vi "Telescope Read Current Status.vi"(8 "error in (no error)":errorcluster, 11 "LDT Telescope in":refnum<class "LDT Telescope.lvclass">) -> (0 "error out":errorcluster, 1 "Raw Response":string="TCS.TCSSharedVariables.TCSHighLevelStatusSV.TCSTcsStatusSV\n<tcsTCSStatus>\n  <tcsVersion>V1.9</tcsVersion>\n  <accessMode>Operator</accessMode>\n  <azCurrentWrap>-1</azCurrentWrap>\n  <heartbeat>15339</heartbeat>\n  <inPositionIsTrue>true</inPositionIsTrue>\n  <m1CoverState>Closed</m1CoverState>\n  <mountGuideMode>OpenLoop</mountGuideMode>\n  <rotCurrentWrap>-1</rotCurrentWrap>\n  <tcsHealth>BAD</tcsHealth>\n  <tcsState>ENABLED</tcsState>\n  <currentTimes>\n    <lst>\n      <hours>22</hours>\n      <minutesTime>32</minutesTime>\n      <secondsTime>33.4</secondsTime>\n    </lst>\n    <time>2023-03-24T17:50:28.166+00:00</time>\n  </currentTimes>\n  <limits>\n    <moonProximity>\n      <distance_deg>85.538145066048</distance_deg>\n      <proximityFlag>false</proximityFlag>\n    </moonProximity>\n    <sunProximity>\n      <distance_deg>101.25098674051</distance_deg>\n      <proximityFlag>false</proximityFlag>\n    </sunProximity>\n    <zenith>\n      <currentZD_deg>66.0067</currentZD_deg>\n      <elZenithLimit_deg>89.3</elZenithLimit_deg>\n      <inBlindSpotIsTrue>false</inBlindSpotIsTrue>\n      <timeToBlindSpot_min>-1</timeToBlindSpot_min>\n      <timeToBlindSpotExit_min>-1</timeToBlindSpotExit_min>\n    </zenith>\n    <airmass>2.4476733769952</airmass>\n    <currentTimeToObservable_min>-1</currentTimeToObservable_min>\n    <currentTimeToUnobservable_min>-1</currentTimeToUnobservable_min>\n    <timeToRotLimit_min>-1</timeToRotLimit_min>\n    <timeToAzLimit_min>-1</timeToAzLimit_min>\n  </limits>\n  <pointingPositions>\n    <azElError>\n      <azError>-0.162</azError>\n      <elError>0.09</elError>\n    </azElError>\n    <currentAzEl>\n      <azimuth>\n        <degreesArc>351</degreesArc>\n        <minutesArc>20</minutesArc>\n        <secondsArc>38.2</secondsArc>\n      </azimuth>\n      <elevation>\n        <degreesAlt>23</degreesAlt>\n        <minutesArc>59</minutesArc>\n        <secondsArc>35.9</secondsArc>\n      </elevation>\n    </currentAzEl>\n    <currentHA>\n      <hours>9</hours>\n      <minutesTime>35</minutesTime>\n      <secondsTime>52.01</secondsTime>\n    </currentHA>\n    <currentRADec>\n      <declination>\n        <degreesDec>77</degreesDec>\n        <minutesArc>5</minutesArc>\n        <secondsArc>36.1</secondsArc>\n      </declination>\n      <equinoxPrefix>J</equinoxPrefix>\n      <equinoxYear>2000</equinoxYear>\n      <frame>FK5</frame>\n      <ra>\n        <hours>12</hours>\n        <minutesTime>55</minutesTime>\n        <secondsTime>53.37</secondsTime>\n      </ra>\n    </currentRADec>\n    <currentParAngle>31.951973490925</currentParAngle>\n    <currentRotatorPositions>\n      <rotPA>322.774092</rotPA>\n      <iaa>185.2</iaa>\n      <rotIPA>0</rotIPA>\n    </currentRotatorPositions>\n    <difftrackStatus>\n      <dAz_ArcsPS>0</dAz_ArcsPS>\n      <dEl_ArcsPS>0</dEl_ArcsPS>\n      <dRA_ArcsPS>0</dRA_ArcsPS>\n      <dDec_ArcsPS>0</dDec_ArcsPS>\n    </difftrackStatus>\n    <objectPA>\n      <EqPA>-0</EqPA>\n      <AzPA>31.951973490925</AzPA>\n    </objectPA>\n    <demandAzEl>\n      <azimuth>\n        <degreesArc>351</degreesArc>\n        <minutesArc>20</minutesArc>\n        <secondsArc>38.68</secondsArc>\n      </azimuth>\n      <elevation>\n        <degreesAlt>23</degreesAlt>\n        <minutesArc>59</minutesArc>\n        <secondsArc>35.61</secondsArc>\n      </elevation>\n    </demandAzEl>\n    <demandRADec>\n      <declination>\n        <degreesDec>77</degreesDec>\n        <minutesArc>5</minutesArc>\n        <secondsArc>36.1</secondsArc>\n      </declination>\n      <equinoxPrefix>J</equinoxPrefix>\n      <equinoxYear>2000</equinoxYear>\n      <frame>FK5</frame>\n      <ra>\n        <hours>12</hours>\n        <minutesTime>55</minutesTime>\n        <secondsTime>53.22</secondsTime>\n      </ra>\n    </demandRADec>\n    <demandRotatorPositions>\n      <rotPA>322.774642</rotPA>\n    </demandRotatorPositions>\n    <targetName>TestTarget</targetName>\n  </pointingPositions>\n  <OffsetStatus>\n    <offsetType>SIMPLE</offsetType>\n    <userOff1>0</userOff1>\n    <userOff2>0</userOff2>\n    <handsetOff1>0</handsetOff1>\n    <handsetOff2>0</handsetOff2>\n  </OffsetStatus>\n  <axesTrackMode>All</axesTrackMode>\n  <inPositionAzIsTrue>true</inPositionAzIsTrue>\n  <inPositionElIsTrue>true</inPositionElIsTrue>\n  <inPositionRotIsTrue>true</inPositionRotIsTrue>\n  <externalTargetCfgCmdPreviewIsTrue>true</externalTargetCfgCmdPreviewIsTrue>\n</tcsTCSStatus>", 2 "Telescope Status":T1, 3 "LDT Telescope out":refnum<class "LDT Telescope.lvclass">, 4 "Cmd Sent":string)   [LabVIEW 2022 SP3, in "LDT Telescope.lvclass"]
uses:
  LDT Telescope.lvclass
  Telescope cluster Status.ctl
  typedefs/CC cluster RA and DEC.ctl
  Telescope enum Status.ctl
  Telescope.lvclass
  LDT Telescope.lvclass/LDT Telescope.ctl
panel:
  out "Timestamp":timestamp
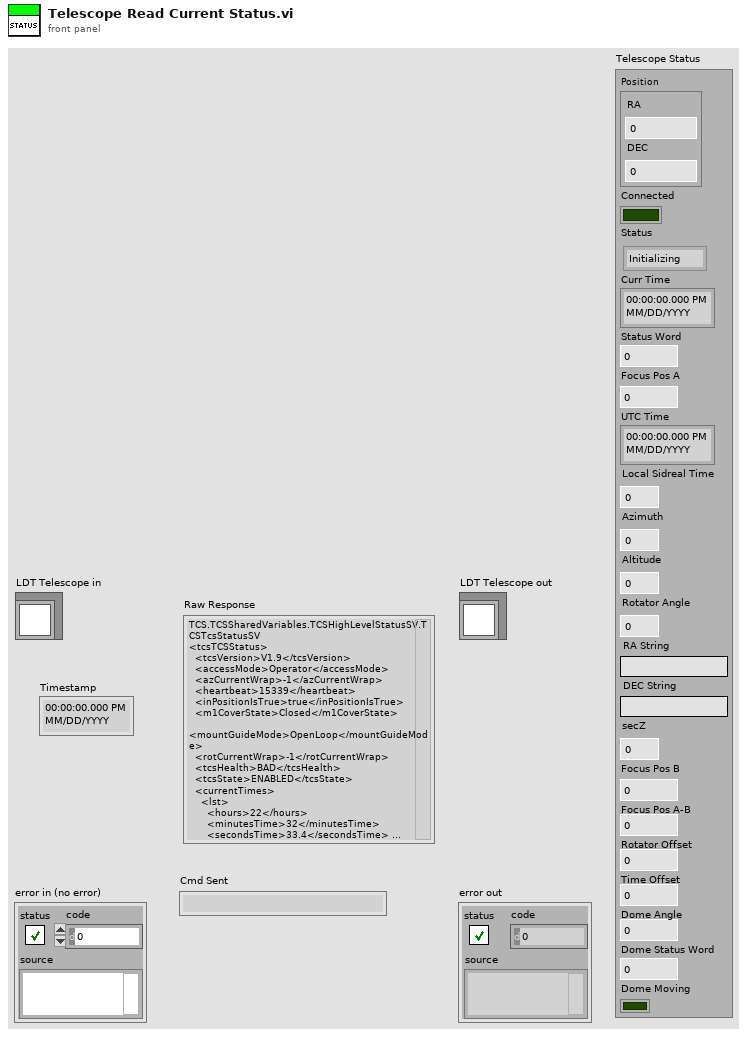
[diagram p1: front panel]
types:
  T1 = typedef "Telescope.lvclass/Telescope cluster Status.ctl" = cluster{"Position":T2, "Connected":bool, "Status":T3, "Curr Time":timestamp, "Status Word":u32, "Focus Pos A":dbl, "UTC Time":timestamp, "Local Sidreal Time":dbl, "Azimuth":dbl, "Altitude":dbl, "Rotator Angle":dbl, "RA String":string, "DEC String":string, "secZ":dbl, "Focus Pos B":dbl, "Focus Pos A-B":dbl, "Rotator Offset":dbl, "Time Offset":dbl, "Dome Angle":dbl, "Dome Status Word":u32, "Dome Moving":bool}
  T2 = typedef "CC cluster RA and DEC.ctl" = cluster{"RA":dbl, "DEC":dbl}
  T3 = typedef "Telescope.lvclass/Telescope enum Status.ctl" = enum16{"Initializing", "Ready", "Moving", "Focusing", "Error"}
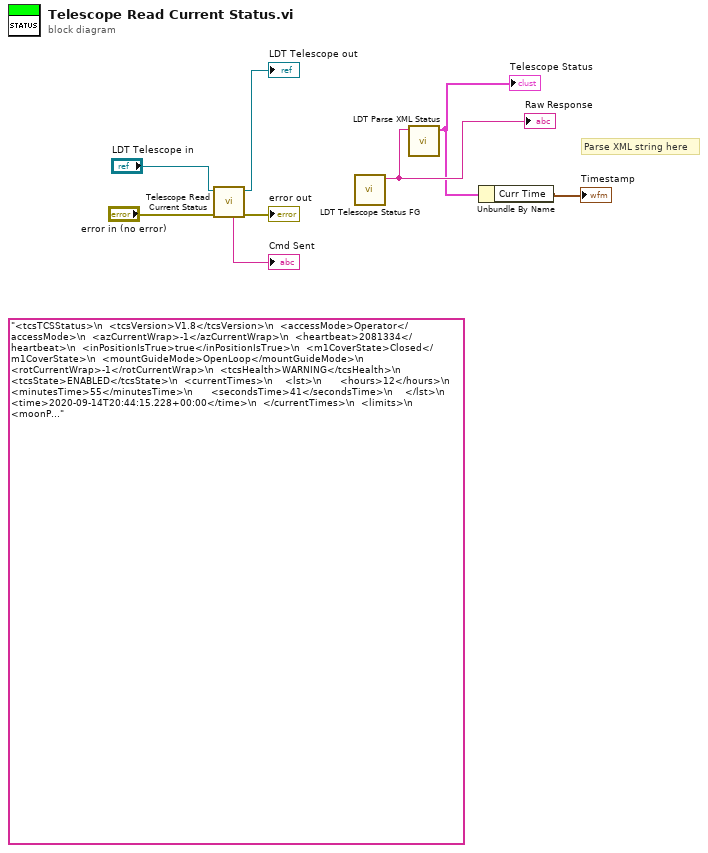
[diagram p0: block diagram]
diagram:
  (unwired) "<tcsTCSStatus>\n  <tcsVersion>V1.8</tcsVersion>\n  <accessMode>Operator</accessMode>\n  <azCurrentWrap>-1</azCurrentWrap>\n  <heartbeat>2081334</heartbeat>\n  <inPositionIsTrue>true</inPositionIsTrue>\n  <m1CoverState>Closed</m1CoverState>\n  <mountGuideMode>OpenLoop</mountGuideMode>\n  <rotCurrentWrap>-1</rotCurrentWrap>\n  <tcsHealth>WARNING</tcsHealth>\n  <tcsState>ENABLED</tcsState>\n  <currentTimes>\n    <lst>\n      <hours>12</hours>\n      <minutesTime>55</minutesTime>\n      <secondsTime>41</secondsTime>\n    </lst>\n    <time>2020-09-14T20:44:15.228+00:00</time>\n  </currentTimes>\n  <limits>\n    <moonProximity>\n      <distance_deg>51.647106572866</distance_deg>\n      <proximityFlag>false</proximityFlag>\n    </moonProximity>\n    <sunProximity>\n      <distance_deg>16.531164188648</distance_deg>\n      <proximityFlag>false</proximityFlag>\n    </sunProximity>\n    <zenith>\n      <currentZD_deg>46.221286</currentZD_deg>\n      <elZenithLimit_deg>89.3</elZenithLimit_deg>\n      <inBlindSpotIsTrue>false</inBlindSpotIsTrue>\n      <timeToBlindSpot_min>-1</timeToBlindSpot_min>\n      <timeToBlindSpotExit_min>-1</timeToBlindSpotExit_min>\n    </zenith>\n    <airmass>1.4438282807451</airmass>\n    <currentTimeToObservable_min>-1</currentTimeToObservable_min>\n    <currentTimeToUnobservable_min>262</currentTimeToUnobservable_min>\n    <timeToRotLimit_min>-1</timeToRotLimit_min>\n    <timeToAzLimit_min>-1</timeToAzLimit_min>\n  </limits>\n  <pointingPositions>\n    <azElError>\n      <azError>-0.9792</azError>\n      <elError>0.1584</elError>\n    </azElError>\n    <currentAzEl>\n      <azimuth>\n        <degreesArc>194</degreesArc>\n        <minutesArc>45</minutesArc>\n        <secondsArc>0.7</secondsArc>\n      </azimuth>\n      <elevation>\n        <degreesAlt>43</degreesAlt>\n        <minutesArc>46</minutesArc>\n        <secondsArc>43.4</secondsArc>\n      </elevation>\n    </currentAzEl>\n    <currentHA>\n      <hours>0</hours>\n      <minutesTime>44</minutesTime>\n      <secondsTime>2.04</secondsTime>\n    </currentHA>\n    <currentRADec>\n      <declination>\n        <degreesDec>-10</degreesDec>\n        <minutesArc>15</minutesArc>\n        <secondsArc>25</secondsArc>\n      </declination>\n      <equinoxPrefix>J</equinoxPrefix>\n      <equinoxYear>2000</equinoxYear>\n      <frame>FK5</frame>\n      <ra>\n        <hours>12</hours>\n        <minutesTime>10</minutesTime>\n        <secondsTime>35.34</secondsTime>\n      </ra>\n    </currentRADec>\n    <currentParAngle>12.557342470137</currentParAngle>\n    <currentRotatorPositions>\n      <rotPA>342.260103</rotPA>\n      <iaa>185.2</iaa>\n      <rotIPA>0</rotIPA>\n    </currentRotatorPositions>\n    <difftrackStatus>\n      <dAz_ArcsPS>0</dAz_ArcsPS>\n      <dEl_ArcsPS>0</dEl_ArcsPS>\n      <dRA_ArcsPS>0</dRA_ArcsPS>\n      <dDec_ArcsPS>0</dDec_ArcsPS>\n    </difftrackStatus>\n    <objectPA>\n      <EqPA>-0</EqPA>\n      <AzPA>12.557342470137</AzPA>\n    </objectPA>\n    <demandAzEl>\n      <azimuth>\n        <degreesArc>194</degreesArc>\n        <minutesArc>45</minutesArc>\n        <secondsArc>3.68</secondsArc>\n      </azimuth>\n      <elevation>\n        <degreesAlt>43</degreesAlt>\n        <minutesArc>46</minutesArc>\n        <secondsArc>42.89</secondsArc>\n      </elevation>\n    </demandAzEl>\n    <demandRADec>\n      <declination>\n        <degreesDec>-10</degreesDec>\n        <minutesArc>15</minutesArc>\n        <secondsArc>25</secondsArc>\n      </declination>\n      <equinoxPrefix>J</equinoxPrefix>\n      <equinoxYear>2000</equinoxYear>\n      <frame>FK5</frame>\n      <ra>\n        <hours>12</hours>\n        <minutesTime>10</minutesTime>\n        <secondsTime>35.24</secondsTime>\n      </ra>\n    </demandRADec>\n    <demandRotatorPositions>\n      <rotPA>342.259442</rotPA>\n    </demandRotatorPositions>\n    <targetName>unspecified</targetName>\n  </pointingPositions>\n  <OffsetStatus>\n    <offsetType>SIMPLE</offsetType>\n    <userOff1>0</userOff1>\n    <userOff2>0</userOff2>\n    <handsetOff1>0</handsetOff1>\n    <handsetOff2>0</handsetOff2>\n  </OffsetStatus>\n  <axesTrackMode>All</axesTrackMode>\n  <inPositionAzIsTrue>true</inPositionAzIsTrue>\n  <inPositionElIsTrue>true</inPositionElIsTrue>\n  <inPositionRotIsTrue>true</inPositionRotIsTrue>\n  <externalTargetCfgCmdPreviewIsTrue>true</externalTargetCfgCmdPreviewIsTrue>\n</tcsTCSStatus>"
  # "Parse XML string here"
  n1 = call-parent "Telescope Read Current Status.vi"("error in (no error)"="error in (no error)", "Telescope in"="LDT Telescope in") -> ("error out"=→"error out":errorcluster, "Telescope out"=→"LDT Telescope out":refnum<class "LDT Telescope.lvclass">, "Cmd Sent"=→"Cmd Sent":string)  [unwired: 5 in, 2 out]
  n2 = call "LDT Telescope Status FG.vi"() -> ("status string out"=w3:string)  [unwired: 10 in, 1 out]
  "Raw Response" <- w3
  n3 = call "LDT Parse XML Status.vi"("XML Status"=w3) -> ("Telescope Status"=w2:T1)  [unwired: 9 in, 1 out]
  "Telescope Status" <- w2
  n4 = Unbundle By Name(w2) -> ("Curr Time"=→"Timestamp":timestamp)
